vi "ReadThrusterMsg.vi"(8 "Error In":errorcluster, 11 "TCPCon In":refnum<k5>) -> (0 "Error Out":errorcluster, 1 "Names":string[](array[string]), 2 "RPM":dbl[](array[numeric]), 3 "TCPCon Out":refnum<k5>, 5 "tau":dbl[](array[numeric]))   [LabVIEW 2014]
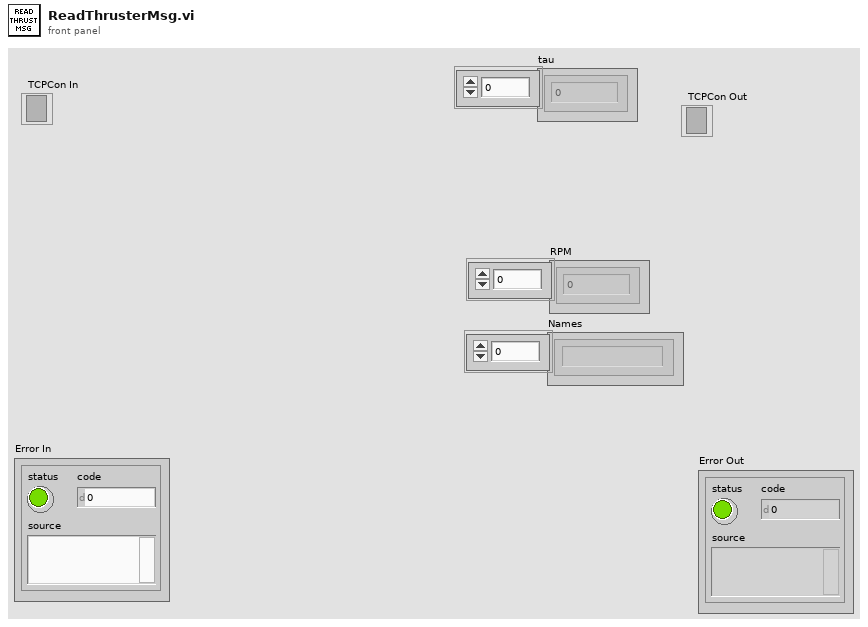
[diagram p1: front panel]
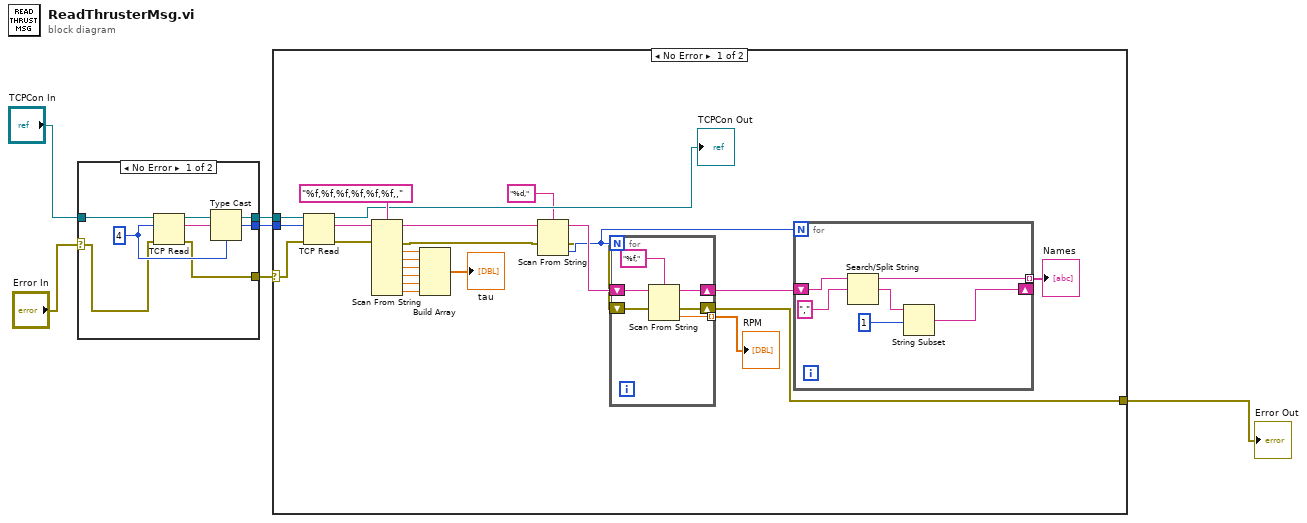
[diagram p0: block diagram]
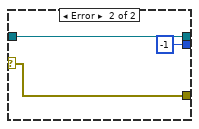
[diagram p2: hidden frame]
diagram:
  n1 = case shown="No Error" "Error In" {
    selector: "Error In" -> [w7 w16]
    tunnel: "TCPCon In" -> [w13 w15]
    tunnel: [w10 -1 ("bytes to read")] -> w5
    tunnel: [w9 w15] -> w4
    tunnel: [w8 w16] -> w3
    frame No Error {
      w11 = 4 ("bytes to read")
      n2 = TCP Read(connection ID=w13, bytes to read=w11, error in (no error)=w7) -> (connection ID out=w9:refnum<k5>, data out=w12:string, error out=w8:errorcluster)  [unwired: 2 in]
      n3 = Type Cast(type=w11, x=w12) -> (*(type *) &x=w10:i32)
    }
    frame Error {
    }
  }
  n4 = case shown="No Error" w3 {
    selector: w3 -> [w21 w53]
    tunnel: w5 -> [w40 _]
    tunnel: w4 -> [w39 _]
    tunnel: [w17 w53] -> w1
    frame No Error {
      n5 = TCP Read(connection ID=w39, bytes to read=w40, error in (no error)=w21) -> (connection ID out=→"TCPCon Out":refnum<k5>, data out=w38:string, error out=w20:errorcluster)  [unwired: 2 in]
      n6 = Scan From String(format string="%f,%f,%f,%f,%f,%f,,", input string=w38, error in=w20) -> (remaining string=w29:string, error out=w19:errorcluster, output 1=w36:dbl, output 2=w35:dbl, output 3=w34:dbl, output 4=w33:dbl, output 5=w32:dbl, output 6=w31:dbl)  [unwired: 7 in, 1 out]
      n7 = Build Array(w36, w35, w34, w33, w32, w31) -> (→"tau":dbl[])
      n8 = Scan From String(format string="%d,", input string=w29, error in=w19) -> (remaining string=w26:string, error out=w18:errorcluster, output 1=w24:i32)  [unwired: 2 in, 1 out]
      n9 = for {
        N: w24 -> [_]
        shift-right: [w51] -> w23
        shift-left: w26 -> [w52]
        tunnel: [w50] -> w25 mode=indexing
        shift-right: [w48] -> w17
        shift-left: w18 -> [w49]
        n10 = Scan From String(format string="%f,", input string=w52, error in=w49) -> (remaining string=w51:string, error out=w48:errorcluster, output 1=w50:dbl)  [unwired: 2 in, 1 out]
      }
      "RPM" <- w25
      n11 = for {
        N: w24 -> [_]
        tunnel: [w45] -> w22 mode=indexing
        shift-right: [w42] -> _
        shift-left: w23 -> [w46]
        n12 = Search/Split String(string=w46, search string/char (-)=",") -> (substring before match=w45:string, match + rest of string=w43:string)  [unwired: 1 in, 1 out]
        n13 = String Subset(string=w43, offset (0)=1) -> (substring=w42:string)  [unwired: 1 in]
      }
      "Names" <- w22
    }
    frame Error {
    }
  }
  "Error Out" <- w1
